vi "wb6OutputPlan.vi"() -> ()   [LabVIEW 2012]
uses:
  <vilib>/addons/database/Auxilliary.llb/DB Tools Cursor Type.ctl
  <vilib>/Utility/NIReport.llb/NI_report.lvclass
  <vilib>/addons/database/Connection.llb/DB Tools Open Connec (Path).vi
  <vilib>/addons/database/Connection.llb/Conn Execute.vi
  <vilib>/addons/database/Recordset.llb/Rec Fetch Recordset Data (R).vi
  <vilib>/addons/database/Recordset.llb/Rec Destroy - Connection.vi
  <vilib>/addons/database/Recordset.llb/Rec Fetch Integer Data (R).vi
  <vilib>/Utility/NIReport.llb/Append Text Table to Report (wrap).vi
  <vilib>/addons/database/_DB Variant To Data/Database Variant To Data.xnode
  <vilib>/addons/database/NI_Database_API.lvlib
  <vilib>/Utility/NIReport.llb/Excel/NI_Excel.lvclass
  <vilib>/addons/_office/NI_ReportGenerationToolkit.lvlib
  <vilib>/Utility/SMTP/NI_SMTPEmail.lvlib
panel:
  out "error out 2":errorcluster
  in  "text data":string[][](array[string])
  in  "text data 2":string[][](array[string])
  out "data 5":string
  out "concatenated string 8":string
  out "concatenated string 7":string
  out "concatenated string 6":string
  out "recordset data 2":variant[][](array[variant])
  out "data 4":string
  out "concatenated string 5":string
  out "error out 3":errorcluster
  out "data 2":string
  out "concatenated string":string
  out "concatenated string 3":string
  out "concatenated string 2":string
  out "recordset data":variant[][](array[variant])
  out "data 3":string
  out "concatenated string 4":string
  out "error out":errorcluster
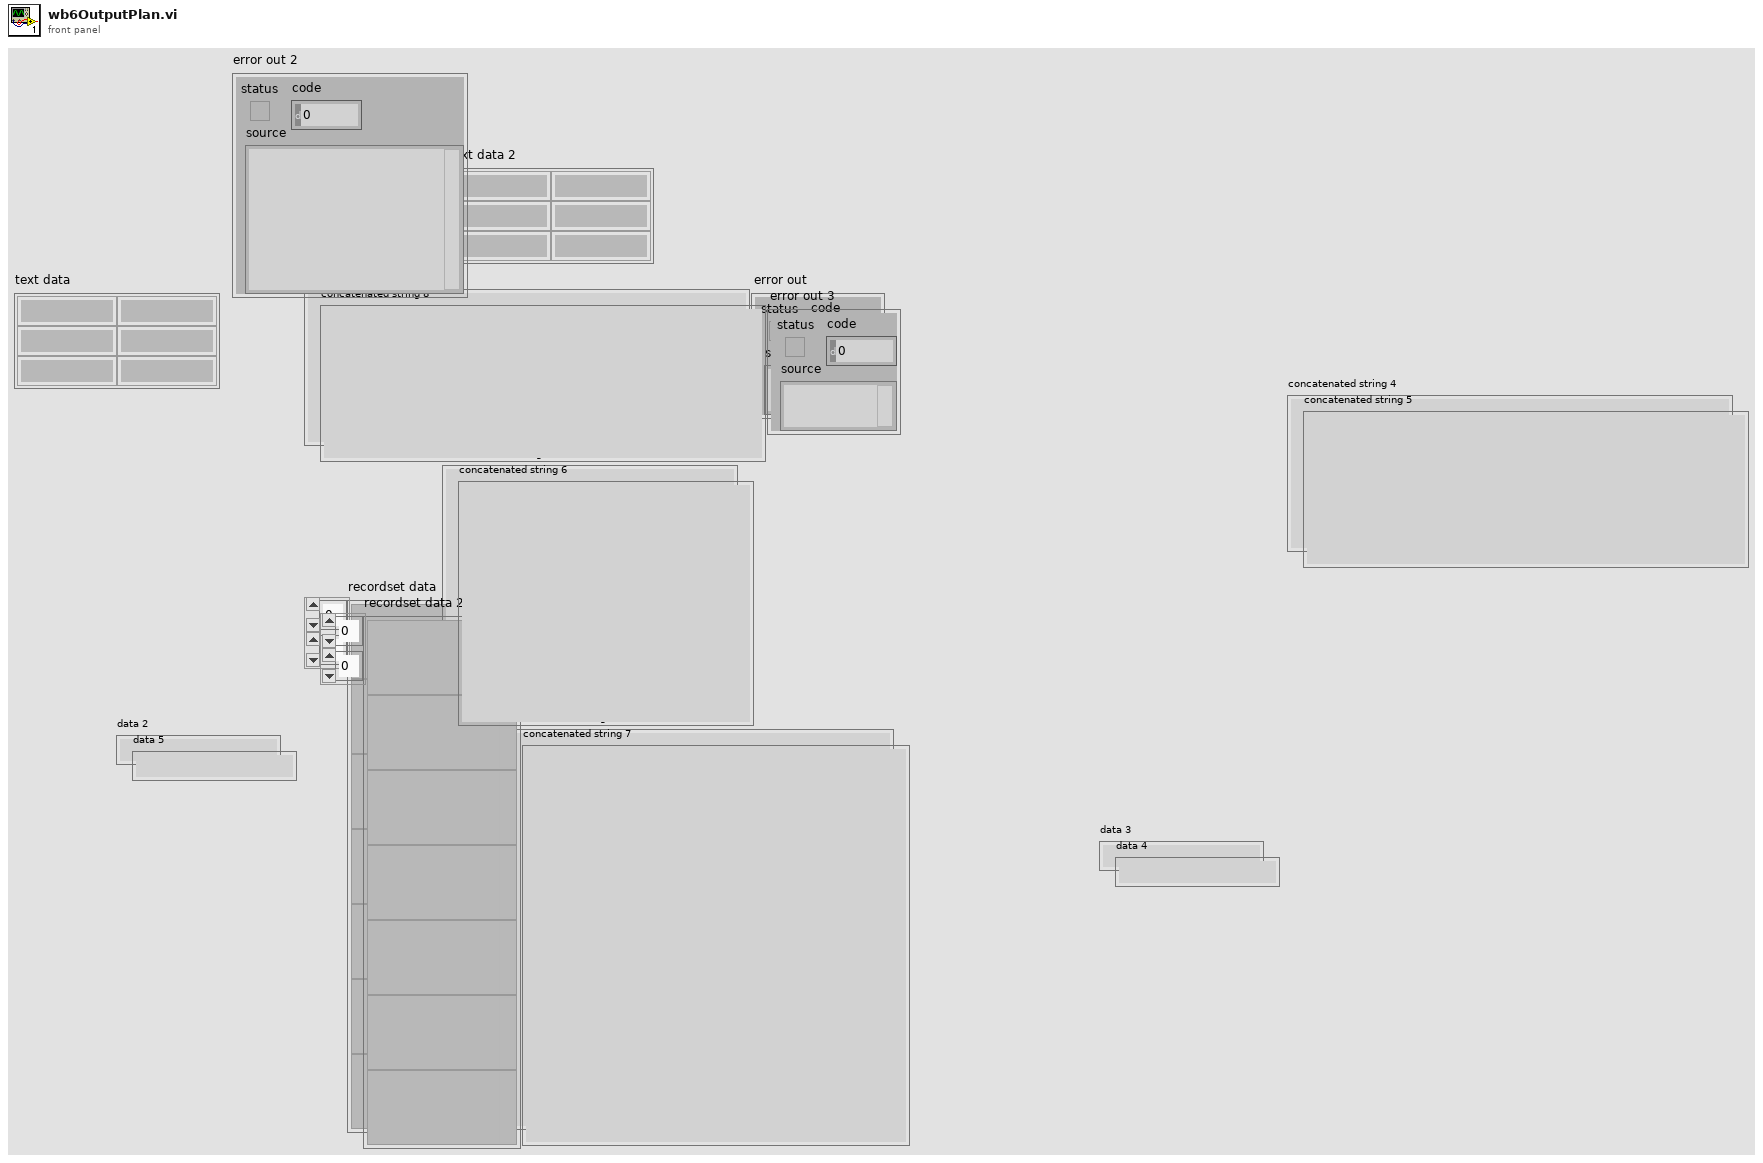
[diagram p1: front panel]
types:
  T1 = typedef "NI_Database_API.lvlib/DB Tools Cursor Type.ctl" = enum16{"forward-only", "keyset", "dynamic", "static"}
  T2 = typedef "NI_Database_API.lvlib/Conn ObjectReference.ctl" = refnum<k1>
  T3 = typedef "NI_Database_API.lvlib/Rec ObjectReference.ctl" = refnum<k1>
  T4 = enum16{"Standard Report", "HTML", "Word", "Excel"}
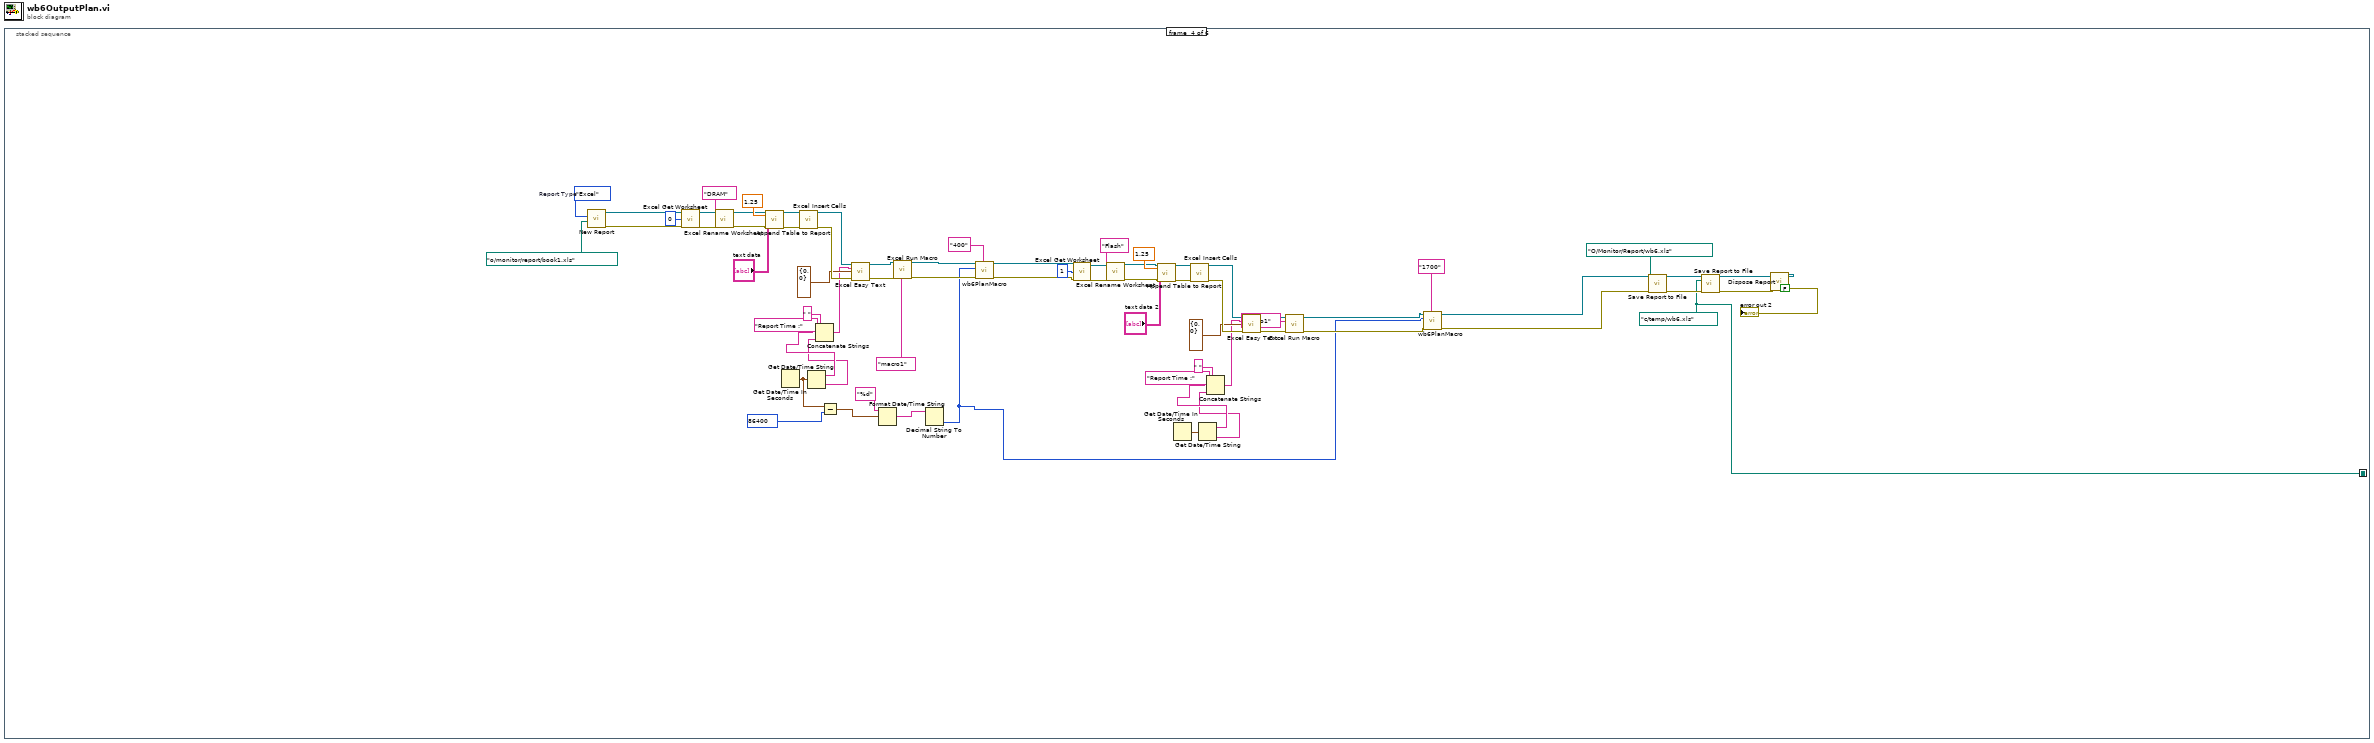
[diagram p0: block diagram]
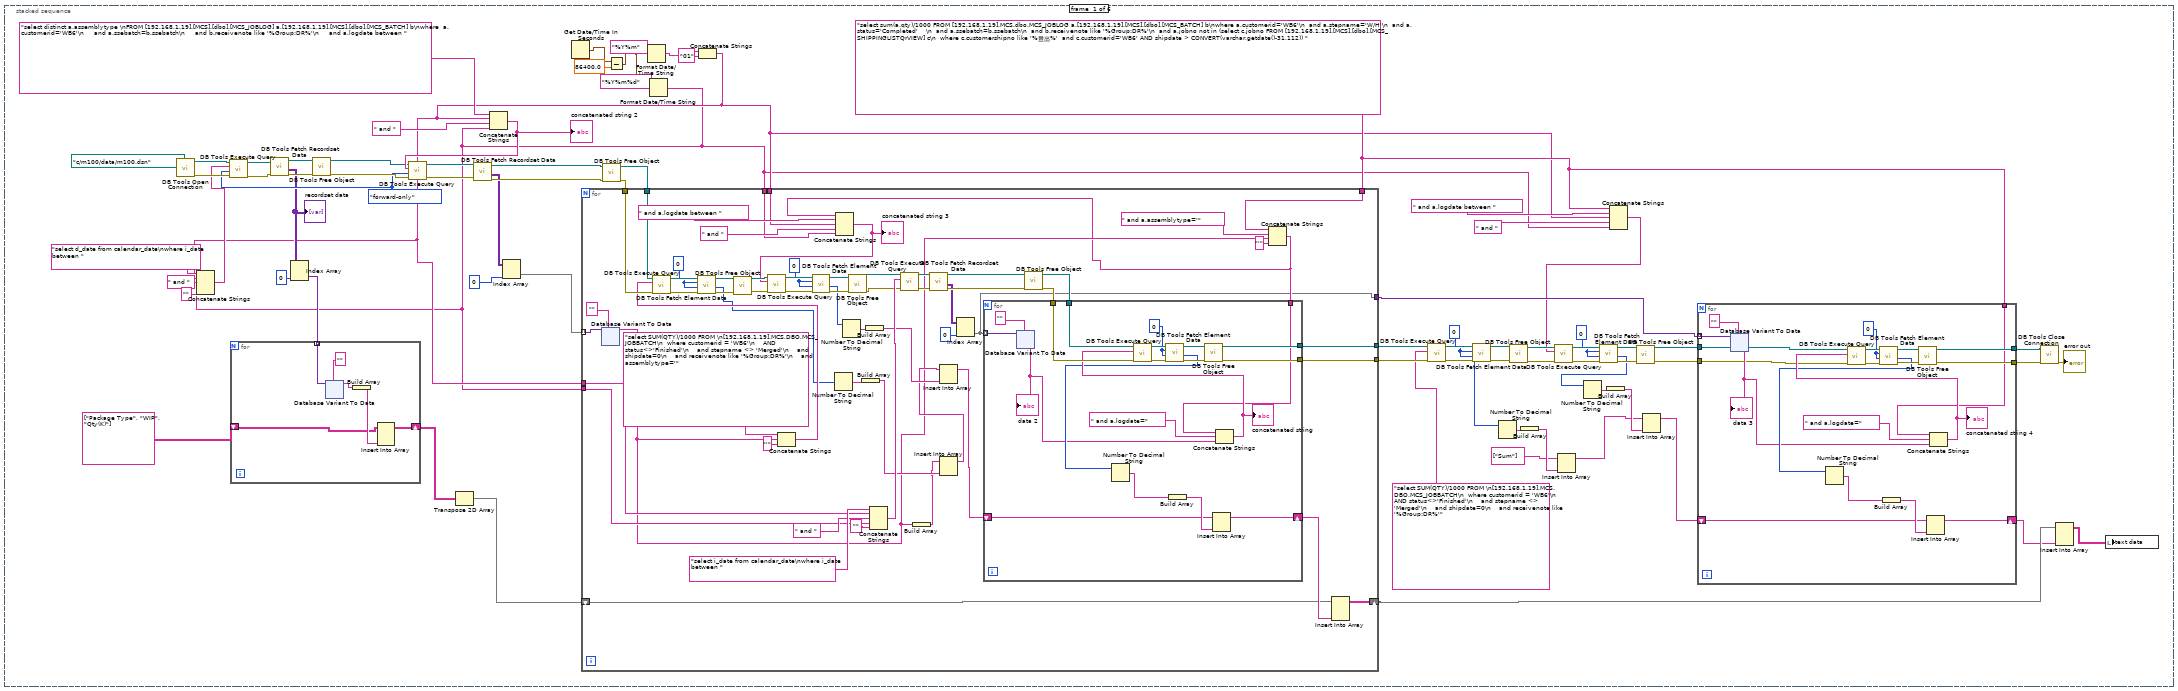
[diagram p2: hidden frame]
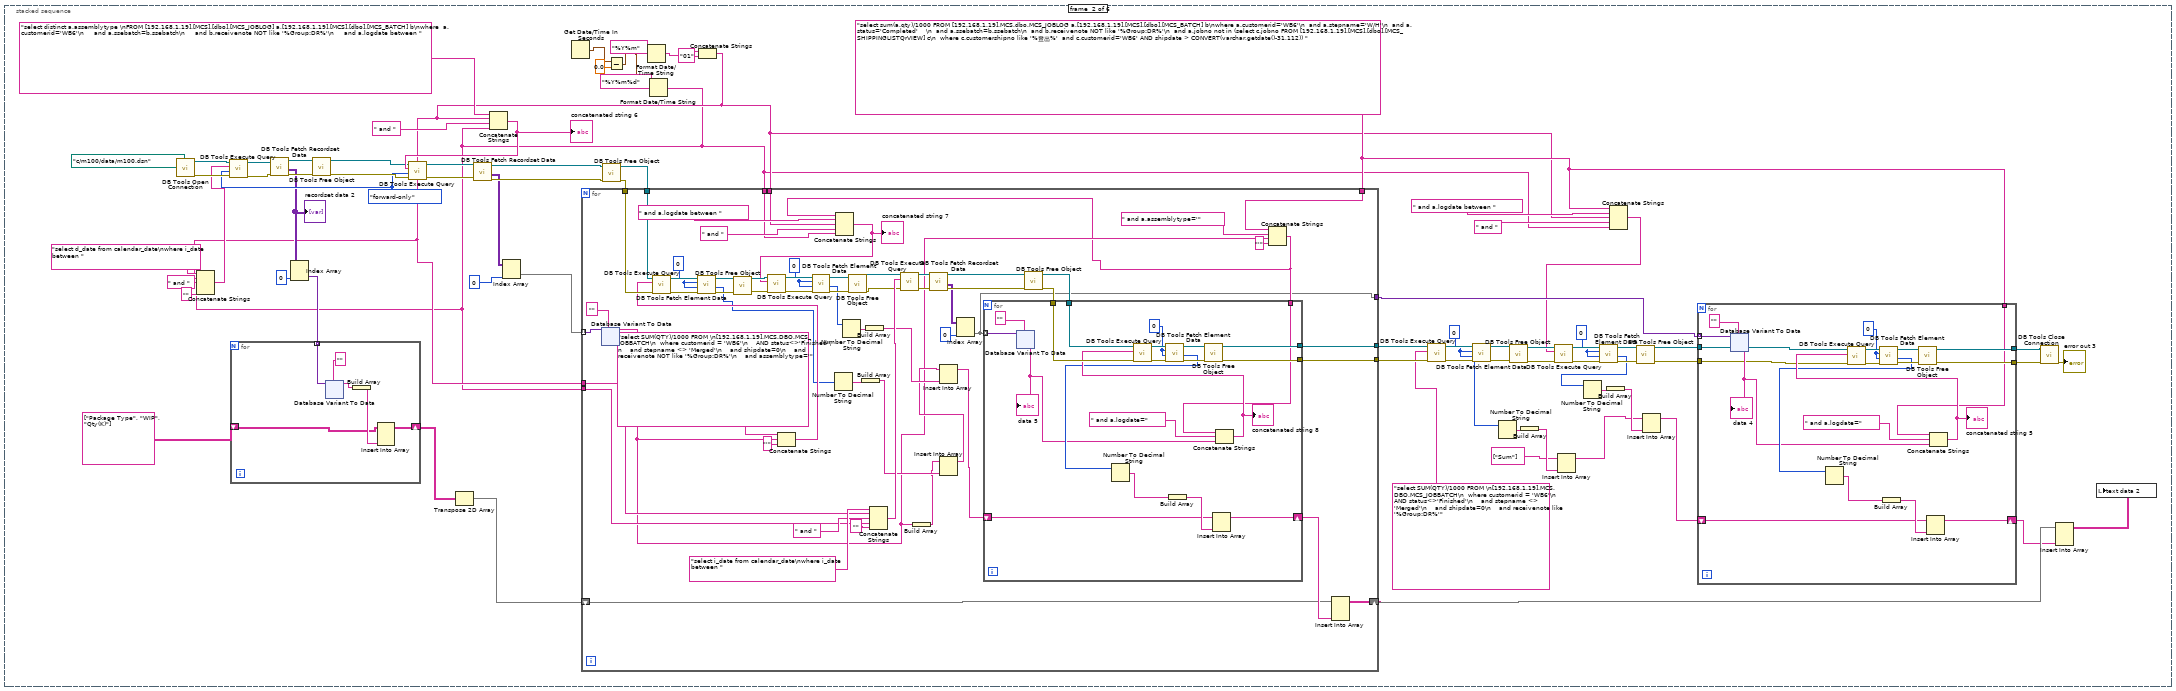
[diagram p3: hidden frame]
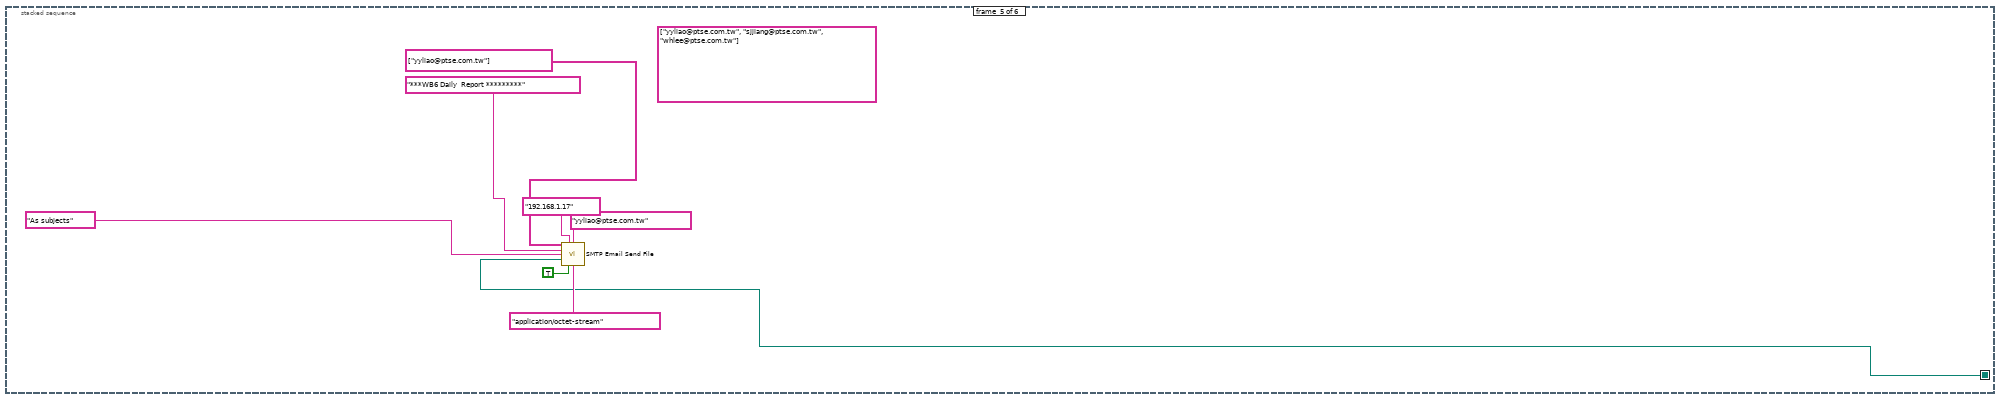
[diagram p5: hidden frame]
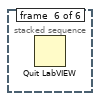
[diagram p6: hidden frame]
diagram:
  n1 = stacked-sequence {
    seq-local: [_ _ _ w641 _ _] -> [_ _ _ _ w697 _]
    frame #0 {
      w17 = 0
      w35 = 0
      w43 = DB_Tools_Cursor_Type."forward-only" ("cursor type")
      w5 = "select sum(a.qty)/1000 FROM [192.168.1.19].MCS.dbo.MCS_JOBLOG a,[192.168.1.19].[MCS].[dbo].[MCS_BATCH] b\nwhere a.customerid='WB6'\n  and a.stepname='W/H'\n  and a.status='Completed'    \n  and a.ssebatch=b.ssebatch\n  and b.receivenote like '%Group:DR%'\n  and a.jobno not in (select c.jobno FROM [192.168.1.19].[MCS].[dbo].[MCS_SHIPPINGLISTQrVIEW] c\n  where c.customershipno like '%登出%'  and c.customerid='WB6' AND shipdate > CONVERT(varchar,getdate()-31,112)) "
      n2 = call-poly <vilib>:"DB Tools Open Connection.vi"("connection information"=path "c:/m100/data/m100.dsn") -> ("error out"=w51:errorcluster, "connection reference"=w55:T2)  [unwired: 7 in]
      n3 = Get Date/Time In Seconds() -> (seconds since 1Jan1904=w68:timestamp)
      n4 = Subtract(x=w68, y=86400.0) -> (x-y=w63:timestamp)
      n5 = Format Date/Time String(time format string (%c)="%Y%m", seconds (now)=w63) -> (date/time string=w66:string)  [unwired: 1 in]
      n6 = Format Date/Time String(time format string (%c)="%Y%m%d", seconds (now)=w63) -> (date/time string=w3:string)  [unwired: 1 in]
      n7 = Concatenate Strings(w66, "01" ("string")) -> (w4:string)
      n8 = Concatenate Strings("select d_date from calendar_date\nwhere i_date between ", w4, " and " ("string"), w3, "" ("string")) -> (w44:string)
      n9 = call-poly <vilib>:"DB Tools Execute Query.vi"("error in (no error)"=w51, "cursor type"=w43, "SQL query"=w44, "connection reference"=w55) -> ("error out"=w50:errorcluster, "recordset reference"=w54:T3)  [unwired: 4 in]
      n10 = call-poly <vilib>:"DB Tools Fetch Recordset Data.vi"("error in (no error)"=w50, "recordset reference"=w54) -> ("error out"=w49:errorcluster, "recordset data"=w42:variant[][], "recordset reference out"=w53:T3)  [unwired: 3 in]
      "recordset data" <- w42
      n11 = Index Array(array=w42, index (col)=0 ("disabled index (col)")) -> (element=w41:variant[])  [unwired: 1 in]
      n12 = for {
        tunnel: w41 -> [w136] mode=indexing
        shift-right: [w132] -> w71
        shift-left: string[][] [["Package Type"], ["WIP"], ["Qty(K)"]] ("array") -> [w131]
        n13 = xnode "Database Variant To Data"("database variant"=w136, "type"="") -> ("data"=w134:string)  [unwired: 1 in, 1 out]
        n14 = Build Array(w134) -> (w133:string[])
        n15 = Insert Into Array(array=w131, new element=w133) -> (w132:string[][])  [unwired: 2 in]
      }
      n16 = call-poly <vilib>:"DB Tools Free Object.vi"("error in (no error)"=w49, "recordset reference"=w53) -> ("error out"=w48:errorcluster, "connection reference"=w52:T2)  [unwired: 8 in]
      n17 = Transpose 2D Array(2D array=w71) -> (transposed array=w70:string[][])
      n18 = Concatenate Strings("select distinct a.assemblytype \nFROM [192.168.1.19].[MCS].[dbo].[MCS_JOBLOG] a,[192.168.1.19].[MCS].[dbo].[MCS_BATCH] b\nwhere  a.customerid='WB6'\n     and a.ssebatch=b.ssebatch\n     and b.receivenote like '%Group:DR%'\n     and a.logdate between ", w4, " and " ("string"), w3) -> (w76:string)
      "concatenated string 2" <- w76
      n19 = call-poly <vilib>:"DB Tools Execute Query.vi"("error in (no error)"=w48, "cursor type"=w43, "SQL query"=w76, "connection reference"=w52) -> ("error out"=w61:errorcluster, "recordset reference"=w62:T3)  [unwired: 4 in]
      n20 = call-poly <vilib>:"DB Tools Fetch Recordset Data.vi"("error in (no error)"=w61, "recordset reference"=w62) -> ("error out"=w77:errorcluster, "recordset data"=w59:variant[][], "recordset reference out"=w78:T3)  [unwired: 3 in]
      n21 = Index Array(array=w59, index (col)=0 ("disabled index (col)")) -> (element=w75:variant[])  [unwired: 1 in]
      n22 = call-poly <vilib>:"DB Tools Free Object.vi"("error in (no error)"=w77, "recordset reference"=w78) -> ("error out"=w73:errorcluster, "connection reference"=w74:T2)  [unwired: 8 in]
      n23 = for {
        tunnel: w75 -> [w227] mode=indexing
        tunnel: w74 -> [w209]
        tunnel: w73 -> [w198]
        tunnel: [w214] -> w34
        tunnel: [w213] -> w33
        tunnel: w4 -> [w221]
        tunnel: w3 -> [w204]
        shift-right: [w211] -> w23
        shift-left: w70 -> [w210]
        tunnel: w5 -> [w177]
        tunnel: w4 -> [w175]
        tunnel: w3 -> [w173]
        tunnel: [w169] -> w27
        w191 = 0
        w201 = 0
        n24 = xnode "Database Variant To Data"("database variant"=w227, "type"="") -> ("data"=w178:string)  [unwired: 1 in, 1 out]
        n25 = Concatenate Strings("select SUM(QTY)/1000 FROM \n[192.168.1.19].MCS.DBO.MCS_JOBBATCH\n  where customerid = 'WB6'\n    AND status<>'Finished'\n    and stepname <> 'Merged'\n    and shipdate=0\n    and receivenote like '%Group:DR%'\n    and assemblytype='" ("SQL query"), w178, "'" ("string")) -> (w197:string)
        n26 = call-poly <vilib>:"DB Tools Execute Query.vi"("error in (no error)"=w198, "SQL query"=w197, "connection reference"=w209) -> ("error out"=w206:errorcluster, "recordset reference"=w208:T3)  [unwired: 5 in]
        n27 = call-poly <vilib>:"DB Tools Fetch Element Data.vi"("error in (no error)"=w206, "type"=w201, "column index"=w201, "recordset reference"=w208) -> ("error out"=w205:errorcluster, "data"=w196:i32, "recordset reference out"=w207:T3)  [unwired: 3 in]
        n28 = call-poly <vilib>:"DB Tools Free Object.vi"("error in (no error)"=w205, "recordset reference"=w207) -> ("error out"=w189:errorcluster, "connection reference"=w190:T2)  [unwired: 8 in]
        n29 = Number To Decimal String(number=w196) -> (decimal integer string=w200:string)  [unwired: 1 in]
        n30 = Build Array(w200) -> (w199:string[])
        n31 = Concatenate Strings("select i_date from calendar_date\nwhere i_date between ", w221, " and " ("string"), w204, "" ("string")) -> (w219:string)
        n32 = Build Array "Build Array"(w178) -> (w180:string[])
        n33 = Insert Into Array(array=w180, new element=w199) -> (w182:string[])  [unwired: 1 in]
        n34 = Concatenate Strings(w177, " and a.assemblytype='" ("string"), w178, "'" ("string")) -> (w171:string)
        n35 = Concatenate Strings(w171, " and a.logdate between " ("string"), w175, " and " ("string"), w173) -> (w172:string)
        "concatenated string 3" <- w172
        n36 = call-poly <vilib>:"DB Tools Execute Query.vi"("error in (no error)"=w189, "SQL query"=w172, "connection reference"=w190) -> ("error out"=w193:errorcluster, "recordset reference"=w195:T3)  [unwired: 5 in]
        n37 = call-poly <vilib>:"DB Tools Fetch Element Data.vi"("error in (no error)"=w193, "type"=w191, "column index"=w191, "recordset reference"=w195) -> ("error out"=w192:errorcluster, "data"=w184:i32, "recordset reference out"=w194:T3)  [unwired: 3 in]
        n38 = Number To Decimal String(number=w184) -> (decimal integer string=w185:string)  [unwired: 1 in]
        n39 = call-poly <vilib>:"DB Tools Free Object.vi"("error in (no error)"=w192, "recordset reference"=w194) -> ("error out"=w187:errorcluster, "connection reference"=w188:T2)  [unwired: 8 in]
        n40 = Build Array(w185) -> (w183:string[])
        n41 = call-poly <vilib>:"DB Tools Execute Query.vi"("error in (no error)"=w187, "SQL query"=w219, "connection reference"=w188) -> ("error out"=w224:errorcluster, "recordset reference"=w226:T3)  [unwired: 5 in]
        n42 = call-poly <vilib>:"DB Tools Fetch Recordset Data.vi"("error in (no error)"=w224, "recordset reference"=w226) -> ("error out"=w223:errorcluster, "recordset data"=w170:variant[][], "recordset reference out"=w225:T3)  [unwired: 3 in]
        n43 = Insert Into Array(array=w182, new element=w183) -> (w181:string[])  [unwired: 1 in]
        n44 = Index Array(array=w170, index (col)=0 ("disabled index (col)")) -> (element=w169:variant[])  [unwired: 1 in]
        n45 = call-poly <vilib>:"DB Tools Free Object.vi"("error in (no error)"=w223, "recordset reference"=w225) -> ("error out"=w215:errorcluster, "connection reference"=w216:T2)  [unwired: 8 in]
        n46 = for {
          tunnel: w169 -> [w248] mode=indexing
          tunnel: w216 -> [w242]
          tunnel: w215 -> [w241]
          tunnel: [w240] -> w214
          tunnel: [w239] -> w213
          shift-right: [w233] -> w212
          shift-left: w181 -> [w232]
          tunnel: w171 -> [w229]
          w236 = 0
          n47 = xnode "Database Variant To Data"("database variant"=w248, "type"="") -> ("data"=w230:string)  [unwired: 1 in, 1 out]
          "data 2" <- w230
          n48 = Concatenate Strings(w229, " and a.logdate=" ("string"), w230) -> (w237:string)
          "concatenated string" <- w237
          n49 = call-poly <vilib>:"DB Tools Execute Query.vi"("error in (no error)"=w241, "SQL query"=w237, "connection reference"=w242) -> ("error out"=w244:errorcluster, "recordset reference"=w246:T3)  [unwired: 5 in]
          n50 = call-poly <vilib>:"DB Tools Fetch Element Data.vi"("error in (no error)"=w244, "type"=w236, "column index"=w236, "recordset reference"=w246) -> ("error out"=w243:errorcluster, "data"=w235:i32, "recordset reference out"=w245:T3)  [unwired: 3 in]
          n51 = Number To Decimal String(number=w235) -> (decimal integer string=w231:string)  [unwired: 1 in]
          n52 = Build Array(w231) -> (w234:string[])
          n53 = call-poly <vilib>:"DB Tools Free Object.vi"("error in (no error)"=w243, "recordset reference"=w245) -> ("error out"=w239:errorcluster, "connection reference"=w240:T2)  [unwired: 8 in]
          n54 = Insert Into Array(array=w232, new element=w234) -> (w233:string[])  [unwired: 1 in]
        }
        n55 = Insert Into Array(array=w210, new element=w212) -> (w211:string[][])  [unwired: 2 in]
      }
      n56 = call-poly <vilib>:"DB Tools Execute Query.vi"("error in (no error)"=w33, "SQL query"="select SUM(QTY)/1000 FROM \n[192.168.1.19].MCS.DBO.MCS_JOBBATCH\n  where customerid = 'WB6'\n    AND status<>'Finished'\n    and stepname <> 'Merged'\n    and shipdate=0\n    and receivenote like '%Group:DR%'", "connection reference"=w34) -> ("error out"=w37:errorcluster, "recordset reference"=w39:T3)  [unwired: 5 in]
      n57 = call-poly <vilib>:"DB Tools Fetch Element Data.vi"("error in (no error)"=w37, "type"=w35, "column index"=w35, "recordset reference"=w39) -> ("error out"=w36:errorcluster, "data"=w30:i32, "recordset reference out"=w38:T3)  [unwired: 3 in]
      n58 = Number To Decimal String(number=w30) -> (decimal integer string=w31:string)  [unwired: 1 in]
      n59 = call-poly <vilib>:"DB Tools Free Object.vi"("error in (no error)"=w36, "recordset reference"=w38) -> ("error out"=w15:errorcluster, "connection reference"=w16:T2)  [unwired: 8 in]
      n60 = Build Array(w31) -> (w29:string[])
      n61 = Insert Into Array(array=string[] ["Sum"], new element=w29) -> (w9:string[])  [unwired: 1 in]
      n62 = Concatenate Strings(w5, " and a.logdate between " ("string"), w4, " and " ("string"), w3) -> (w2:string)
      n63 = call-poly <vilib>:"DB Tools Execute Query.vi"("error in (no error)"=w15, "SQL query"=w2, "connection reference"=w16) -> ("error out"=w19:errorcluster, "recordset reference"=w21:T3)  [unwired: 5 in]
      n64 = call-poly <vilib>:"DB Tools Fetch Element Data.vi"("error in (no error)"=w19, "type"=w17, "column index"=w17, "recordset reference"=w21) -> ("error out"=w18:errorcluster, "data"=w10:i32, "recordset reference out"=w20:T3)  [unwired: 3 in]
      n65 = Number To Decimal String(number=w10) -> (decimal integer string=w12:string)  [unwired: 1 in]
      n66 = Build Array(w12) -> (w11:string[])
      n67 = call-poly <vilib>:"DB Tools Free Object.vi"("error in (no error)"=w18, "recordset reference"=w20) -> ("error out"=w13:errorcluster, "connection reference"=w14:T2)  [unwired: 8 in]
      n68 = Insert Into Array(array=w9, new element=w11) -> (w8:string[])  [unwired: 1 in]
      n69 = for {
        tunnel: w27 -> [w81] mode=indexing
        tunnel: [w93] -> w26
        tunnel: [w92] -> w25
        shift-right: [w86] -> w22
        shift-left: w8 -> [w85]
        tunnel: w5 -> [w82]
        tunnel: w14 -> [w80]
        tunnel: w13 -> [w79]
        w89 = 0
        n70 = xnode "Database Variant To Data"("database variant"=w81, "type"="") -> ("data"=w83:string)  [unwired: 1 in, 1 out]
        "data 3" <- w83
        n71 = Concatenate Strings(w82, " and a.logdate=" ("string"), w83) -> (w90:string)
        "concatenated string 4" <- w90
        n72 = call-poly <vilib>:"DB Tools Execute Query.vi"("error in (no error)"=w79, "SQL query"=w90, "connection reference"=w80) -> ("error out"=w95:errorcluster, "recordset reference"=w97:T3)  [unwired: 5 in]
        n73 = call-poly <vilib>:"DB Tools Fetch Element Data.vi"("error in (no error)"=w95, "type"=w89, "column index"=w89, "recordset reference"=w97) -> ("error out"=w94:errorcluster, "data"=w88:i32, "recordset reference out"=w96:T3)  [unwired: 3 in]
        n74 = Number To Decimal String(number=w88) -> (decimal integer string=w84:string)  [unwired: 1 in]
        n75 = Build Array(w84) -> (w87:string[])
        n76 = call-poly <vilib>:"DB Tools Free Object.vi"("error in (no error)"=w94, "recordset reference"=w96) -> ("error out"=w92:errorcluster, "connection reference"=w93:T2)  [unwired: 8 in]
        n77 = Insert Into Array(array=w85, new element=w87) -> (w86:string[])  [unwired: 1 in]
      }
      n78 = call <vilib>:"DB Tools Close Connection.vi"("error in (no error)"=w25, "connection reference"=w26) -> ("error out"=→"error out":errorcluster)  [unwired: 5 in]
      n79 = Insert Into Array(array=w23, new element=w22) -> (w1:string[][])  [unwired: 2 in]
      n80 = local write "text data"(w1) -> ()
    }
    frame #1 {
      w329 = 0
      w347 = 0
      w355 = DB_Tools_Cursor_Type."forward-only" ("cursor type")
      w317 = "select sum(a.qty)/1000 FROM [192.168.1.19].MCS.dbo.MCS_JOBLOG a,[192.168.1.19].[MCS].[dbo].[MCS_BATCH] b\nwhere a.customerid='WB6'\n  and a.stepname='W/H'\n  and a.status='Completed'    \n  and a.ssebatch=b.ssebatch\n  and b.receivenote NOT like '%Group:DR%'\n  and a.jobno not in (select c.jobno FROM [192.168.1.19].[MCS].[dbo].[MCS_SHIPPINGLISTQrVIEW] c\n  where c.customershipno like '%登出%'  and c.customerid='WB6' AND shipdate > CONVERT(varchar,getdate()-31,112)) "
      n81 = call-poly <vilib>:"DB Tools Open Connection.vi"("connection information"=path "c:/m100/data/m100.dsn") -> ("error out"=w363:errorcluster, "connection reference"=w367:T2)  [unwired: 7 in]
      n82 = Get Date/Time In Seconds() -> (seconds since 1Jan1904=w380:timestamp)
      n83 = Subtract(x=w380, y=0.0) -> (x-y=w375:timestamp)
      n84 = Format Date/Time String(time format string (%c)="%Y%m", seconds (now)=w375) -> (date/time string=w378:string)  [unwired: 1 in]
      n85 = Format Date/Time String(time format string (%c)="%Y%m%d", seconds (now)=w375) -> (date/time string=w315:string)  [unwired: 1 in]
      n86 = Concatenate Strings(w378, "01" ("string")) -> (w316:string)
      n87 = Concatenate Strings("select d_date from calendar_date\nwhere i_date between ", w316, " and " ("string"), w315, "" ("string")) -> (w356:string)
      n88 = call-poly <vilib>:"DB Tools Execute Query.vi"("error in (no error)"=w363, "cursor type"=w355, "SQL query"=w356, "connection reference"=w367) -> ("error out"=w362:errorcluster, "recordset reference"=w366:T3)  [unwired: 4 in]
      n89 = call-poly <vilib>:"DB Tools Fetch Recordset Data.vi"("error in (no error)"=w362, "recordset reference"=w366) -> ("error out"=w361:errorcluster, "recordset data"=w354:variant[][], "recordset reference out"=w365:T3)  [unwired: 3 in]
      "recordset data 2" <- w354
      n90 = Index Array(array=w354, index (col)=0 ("disabled index (col)")) -> (element=w353:variant[])  [unwired: 1 in]
      n91 = for {
        tunnel: w353 -> [w448] mode=indexing
        shift-right: [w444] -> w383
        shift-left: string[][] [["Package Type"], ["WIP"], ["Qty(K)"]] ("array") -> [w443]
        n92 = xnode "Database Variant To Data"("database variant"=w448, "type"="") -> ("data"=w446:string)  [unwired: 1 in, 1 out]
        n93 = Build Array(w446) -> (w445:string[])
        n94 = Insert Into Array(array=w443, new element=w445) -> (w444:string[][])  [unwired: 2 in]
      }
      n95 = call-poly <vilib>:"DB Tools Free Object.vi"("error in (no error)"=w361, "recordset reference"=w365) -> ("error out"=w360:errorcluster, "connection reference"=w364:T2)  [unwired: 8 in]
      n96 = Transpose 2D Array(2D array=w383) -> (transposed array=w382:string[][])
      n97 = Concatenate Strings("select distinct a.assemblytype \nFROM [192.168.1.19].[MCS].[dbo].[MCS_JOBLOG] a,[192.168.1.19].[MCS].[dbo].[MCS_BATCH] b\nwhere  a.customerid='WB6'\n     and a.ssebatch=b.ssebatch\n     and b.receivenote NOT like '%Group:DR%'\n     and a.logdate between ", w316, " and " ("string"), w315) -> (w388:string)
      "concatenated string 6" <- w388
      n98 = call-poly <vilib>:"DB Tools Execute Query.vi"("error in (no error)"=w360, "cursor type"=w355, "SQL query"=w388, "connection reference"=w364) -> ("error out"=w373:errorcluster, "recordset reference"=w374:T3)  [unwired: 4 in]
      n99 = call-poly <vilib>:"DB Tools Fetch Recordset Data.vi"("error in (no error)"=w373, "recordset reference"=w374) -> ("error out"=w389:errorcluster, "recordset data"=w371:variant[][], "recordset reference out"=w390:T3)  [unwired: 3 in]
      n100 = Index Array(array=w371, index (col)=0 ("disabled index (col)")) -> (element=w387:variant[])  [unwired: 1 in]
      n101 = call-poly <vilib>:"DB Tools Free Object.vi"("error in (no error)"=w389, "recordset reference"=w390) -> ("error out"=w385:errorcluster, "connection reference"=w386:T2)  [unwired: 8 in]
      n102 = for {
        tunnel: w387 -> [w539] mode=indexing
        tunnel: w386 -> [w521]
        tunnel: w385 -> [w510]
        tunnel: [w526] -> w346
        tunnel: [w525] -> w345
        tunnel: w316 -> [w533]
        tunnel: w315 -> [w516]
        shift-right: [w523] -> w335
        shift-left: w382 -> [w522]
        tunnel: w317 -> [w489]
        tunnel: w316 -> [w487]
        tunnel: w315 -> [w485]
        tunnel: [w481] -> w339
        w503 = 0
        w513 = 0
        n103 = xnode "Database Variant To Data"("database variant"=w539, "type"="") -> ("data"=w490:string)  [unwired: 1 in, 1 out]
        n104 = Concatenate Strings("select SUM(QTY)/1000 FROM \n[192.168.1.19].MCS.DBO.MCS_JOBBATCH\n  where customerid = 'WB6'\n    AND status<>'Finished'\n    and stepname <> 'Merged'\n    and shipdate=0\n    and receivenote NOT like '%Group:DR%'\n    and assemblytype='" ("SQL query"), w490, "'" ("string")) -> (w509:string)
        n105 = call-poly <vilib>:"DB Tools Execute Query.vi"("error in (no error)"=w510, "SQL query"=w509, "connection reference"=w521) -> ("error out"=w518:errorcluster, "recordset reference"=w520:T3)  [unwired: 5 in]
        n106 = call-poly <vilib>:"DB Tools Fetch Element Data.vi"("error in (no error)"=w518, "type"=w513, "column index"=w513, "recordset reference"=w520) -> ("error out"=w517:errorcluster, "data"=w508:i32, "recordset reference out"=w519:T3)  [unwired: 3 in]
        n107 = call-poly <vilib>:"DB Tools Free Object.vi"("error in (no error)"=w517, "recordset reference"=w519) -> ("error out"=w501:errorcluster, "connection reference"=w502:T2)  [unwired: 8 in]
        n108 = Number To Decimal String(number=w508) -> (decimal integer string=w512:string)  [unwired: 1 in]
        n109 = Build Array(w512) -> (w511:string[])
        n110 = Concatenate Strings("select i_date from calendar_date\nwhere i_date between ", w533, " and " ("string"), w516, "" ("string")) -> (w531:string)
        n111 = Build Array "Build Array"(w490) -> (w492:string[])
        n112 = Insert Into Array(array=w492, new element=w511) -> (w494:string[])  [unwired: 1 in]
        n113 = Concatenate Strings(w489, " and a.assemblytype='" ("string"), w490, "'" ("string")) -> (w483:string)
        n114 = Concatenate Strings(w483, " and a.logdate between " ("string"), w487, " and " ("string"), w485) -> (w484:string)
        "concatenated string 7" <- w484
        n115 = call-poly <vilib>:"DB Tools Execute Query.vi"("error in (no error)"=w501, "SQL query"=w484, "connection reference"=w502) -> ("error out"=w505:errorcluster, "recordset reference"=w507:T3)  [unwired: 5 in]
        n116 = call-poly <vilib>:"DB Tools Fetch Element Data.vi"("error in (no error)"=w505, "type"=w503, "column index"=w503, "recordset reference"=w507) -> ("error out"=w504:errorcluster, "data"=w496:i32, "recordset reference out"=w506:T3)  [unwired: 3 in]
        n117 = Number To Decimal String(number=w496) -> (decimal integer string=w497:string)  [unwired: 1 in]
        n118 = call-poly <vilib>:"DB Tools Free Object.vi"("error in (no error)"=w504, "recordset reference"=w506) -> ("error out"=w499:errorcluster, "connection reference"=w500:T2)  [unwired: 8 in]
        n119 = Build Array(w497) -> (w495:string[])
        n120 = call-poly <vilib>:"DB Tools Execute Query.vi"("error in (no error)"=w499, "SQL query"=w531, "connection reference"=w500) -> ("error out"=w536:errorcluster, "recordset reference"=w538:T3)  [unwired: 5 in]
        n121 = call-poly <vilib>:"DB Tools Fetch Recordset Data.vi"("error in (no error)"=w536, "recordset reference"=w538) -> ("error out"=w535:errorcluster, "recordset data"=w482:variant[][], "recordset reference out"=w537:T3)  [unwired: 3 in]
        n122 = Insert Into Array(array=w494, new element=w495) -> (w493:string[])  [unwired: 1 in]
        n123 = Index Array(array=w482, index (col)=0 ("disabled index (col)")) -> (element=w481:variant[])  [unwired: 1 in]
        n124 = call-poly <vilib>:"DB Tools Free Object.vi"("error in (no error)"=w535, "recordset reference"=w537) -> ("error out"=w527:errorcluster, "connection reference"=w528:T2)  [unwired: 8 in]
        n125 = for {
          tunnel: w481 -> [w560] mode=indexing
          tunnel: w528 -> [w554]
          tunnel: w527 -> [w553]
          tunnel: [w552] -> w526
          tunnel: [w551] -> w525
          shift-right: [w545] -> w524
          shift-left: w493 -> [w544]
          tunnel: w483 -> [w541]
          w548 = 0
          n126 = xnode "Database Variant To Data"("database variant"=w560, "type"="") -> ("data"=w542:string)  [unwired: 1 in, 1 out]
          "data 5" <- w542
          n127 = Concatenate Strings(w541, " and a.logdate=" ("string"), w542) -> (w549:string)
          "concatenated string 8" <- w549
          n128 = call-poly <vilib>:"DB Tools Execute Query.vi"("error in (no error)"=w553, "SQL query"=w549, "connection reference"=w554) -> ("error out"=w556:errorcluster, "recordset reference"=w558:T3)  [unwired: 5 in]
          n129 = call-poly <vilib>:"DB Tools Fetch Element Data.vi"("error in (no error)"=w556, "type"=w548, "column index"=w548, "recordset reference"=w558) -> ("error out"=w555:errorcluster, "data"=w547:i32, "recordset reference out"=w557:T3)  [unwired: 3 in]
          n130 = Number To Decimal String(number=w547) -> (decimal integer string=w543:string)  [unwired: 1 in]
          n131 = Build Array(w543) -> (w546:string[])
          n132 = call-poly <vilib>:"DB Tools Free Object.vi"("error in (no error)"=w555, "recordset reference"=w557) -> ("error out"=w551:errorcluster, "connection reference"=w552:T2)  [unwired: 8 in]
          n133 = Insert Into Array(array=w544, new element=w546) -> (w545:string[])  [unwired: 1 in]
        }
        n134 = Insert Into Array(array=w522, new element=w524) -> (w523:string[][])  [unwired: 2 in]
      }
      n135 = call-poly <vilib>:"DB Tools Execute Query.vi"("error in (no error)"=w345, "SQL query"="select SUM(QTY)/1000 FROM \n[192.168.1.19].MCS.DBO.MCS_JOBBATCH\n  where customerid = 'WB6'\n    AND status<>'Finished'\n    and stepname <> 'Merged'\n    and shipdate=0\n    and receivenote like '%Group:DR%'", "connection reference"=w346) -> ("error out"=w349:errorcluster, "recordset reference"=w351:T3)  [unwired: 5 in]
      n136 = call-poly <vilib>:"DB Tools Fetch Element Data.vi"("error in (no error)"=w349, "type"=w347, "column index"=w347, "recordset reference"=w351) -> ("error out"=w348:errorcluster, "data"=w342:i32, "recordset reference out"=w350:T3)  [unwired: 3 in]
      n137 = Number To Decimal String(number=w342) -> (decimal integer string=w343:string)  [unwired: 1 in]
      n138 = call-poly <vilib>:"DB Tools Free Object.vi"("error in (no error)"=w348, "recordset reference"=w350) -> ("error out"=w327:errorcluster, "connection reference"=w328:T2)  [unwired: 8 in]
      n139 = Build Array(w343) -> (w341:string[])
      n140 = Insert Into Array(array=string[] ["Sum"], new element=w341) -> (w321:string[])  [unwired: 1 in]
      n141 = Concatenate Strings(w317, " and a.logdate between " ("string"), w316, " and " ("string"), w315) -> (w314:string)
      n142 = call-poly <vilib>:"DB Tools Execute Query.vi"("error in (no error)"=w327, "SQL query"=w314, "connection reference"=w328) -> ("error out"=w331:errorcluster, "recordset reference"=w333:T3)  [unwired: 5 in]
      n143 = call-poly <vilib>:"DB Tools Fetch Element Data.vi"("error in (no error)"=w331, "type"=w329, "column index"=w329, "recordset reference"=w333) -> ("error out"=w330:errorcluster, "data"=w322:i32, "recordset reference out"=w332:T3)  [unwired: 3 in]
      n144 = Number To Decimal String(number=w322) -> (decimal integer string=w324:string)  [unwired: 1 in]
      n145 = Build Array(w324) -> (w323:string[])
      n146 = call-poly <vilib>:"DB Tools Free Object.vi"("error in (no error)"=w330, "recordset reference"=w332) -> ("error out"=w325:errorcluster, "connection reference"=w326:T2)  [unwired: 8 in]
      n147 = Insert Into Array(array=w321, new element=w323) -> (w320:string[])  [unwired: 1 in]
      n148 = for {
        tunnel: w339 -> [w393] mode=indexing
        tunnel: [w405] -> w338
        tunnel: [w404] -> w337
        shift-right: [w398] -> w334
        shift-left: w320 -> [w397]
        tunnel: w317 -> [w394]
        tunnel: w326 -> [w392]
        tunnel: w325 -> [w391]
        w401 = 0
        n149 = xnode "Database Variant To Data"("database variant"=w393, "type"="") -> ("data"=w395:string)  [unwired: 1 in, 1 out]
        "data 4" <- w395
        n150 = Concatenate Strings(w394, " and a.logdate=" ("string"), w395) -> (w402:string)
        "concatenated string 5" <- w402
        n151 = call-poly <vilib>:"DB Tools Execute Query.vi"("error in (no error)"=w391, "SQL query"=w402, "connection reference"=w392) -> ("error out"=w407:errorcluster, "recordset reference"=w409:T3)  [unwired: 5 in]
        n152 = call-poly <vilib>:"DB Tools Fetch Element Data.vi"("error in (no error)"=w407, "type"=w401, "column index"=w401, "recordset reference"=w409) -> ("error out"=w406:errorcluster, "data"=w400:i32, "recordset reference out"=w408:T3)  [unwired: 3 in]
        n153 = Number To Decimal String(number=w400) -> (decimal integer string=w396:string)  [unwired: 1 in]
        n154 = Build Array(w396) -> (w399:string[])
        n155 = call-poly <vilib>:"DB Tools Free Object.vi"("error in (no error)"=w406, "recordset reference"=w408) -> ("error out"=w404:errorcluster, "connection reference"=w405:T2)  [unwired: 8 in]
        n156 = Insert Into Array(array=w397, new element=w399) -> (w398:string[])  [unwired: 1 in]
      }
      n157 = call <vilib>:"DB Tools Close Connection.vi"("error in (no error)"=w337, "connection reference"=w338) -> ("error out"=→"error out 3":errorcluster)  [unwired: 5 in]
      n158 = Insert Into Array(array=w335, new element=w334) -> (w313:string[][])  [unwired: 2 in]
      n159 = local write "text data 2"(w313) -> ()
    }
    frame #2 {
      # "select a.customerid,a.assemblytype,a.producttype,a.jobno,a.qty,a.logdate,a.logtime FROM [192.168.1.19].MCS.dbo.MCS_JOBLOG a,[192.168.1.19].[MCS].[dbo].[MCS_BATCH] b\nwhere a.customerid='WB6'\n  and a.stepname='W/H'\n  and a.status='Completed'    \n  and a.ssebatch=b.ssebatch\n  and b.receivenote NOT like '%Group:DR%'\n  and a.jobno not in (select c.jobno FROM [192.168.1.19].[MCS].[dbo].[MCS_SHIPPINGLISTQrVIEW] c\n  where c.customershipno like '%登出%'  and c.customerid='WB6' AND shipdate > CONVERT(varchar,getdate()-31,112)) \n  and a.logdate =20150921"
    }
    frame #3 {
      w641 = path "c:/temp/wb6.xls" ("report file path")
      w695 = T4."Excel"  # Report Type
      n160 = call <vilib>:"New Report.vi"("report type"=w695, "template (empty)"=path "o:/monitor/report/book1.xls" ("Report Template")) -> ("report out"=w690:refnum<class "NI_report.lvclass">, "error out"=w689:errorcluster)  [unwired: 12 in]
      n161 = call <vilib>:"Excel Get Worksheet.vi"("report in"=w690, "worksheet index (0)"=0, "error in (no error)"=w689) -> ("report out"=w687:refnum<class "NI_report.lvclass">, "error out"=w685:errorcluster)  [unwired: 11 in]
      n162 = call <vilib>:"Excel Rename Worksheet.vi"("report in"=w687, "worksheet name (\"\")"="DRAM" ("worksheet name (\"\")"), "error in (no error)"=w685) -> ("report out"=w686:refnum<class "NI_report.lvclass">, "error out"=w684:errorcluster)  [unwired: 11 in]
      n163 = call-poly <vilib>:"Append Table to Report.vi"("report in"=w686, "column width (1)"=1.25, "text data"="text data", "error in (no error)"=w684) -> ("report out"=w692:refnum<class "NI_report.lvclass">, "error out"=w691:errorcluster)  [unwired: 8 in, 2 out]
      n164 = Get Date/Time In Seconds() -> (seconds since 1Jan1904=w635:timestamp)
      n165 = call <vilib>:"Excel Insert Cells.vi"("report in"=w692, "error in (no error)"=w691) -> ("report out"=w682:refnum<class "NI_report.lvclass">, "error out"=w681:errorcluster)  [unwired: 12 in]
      n166 = Get Date/Time String(seconds (now)=w635) -> (date string=w678:string, time string=w676:string)  [unwired: 2 in]
      n167 = Concatenate Strings("Report Time :" ("string"), w678, " " ("string"), w676) -> (w675:string)
      n168 = Subtract(x=w635, y=86400) -> (x-y=w633:timestamp)
      n169 = call <vilib>:"Excel Easy Text.vi"("report in"=w682, "text"=w675, "start (-1, -1)"=cluster{"row":i32, "column":i32} {"row"=0, "column"=0} ("end (-1, -1)"), "error in (no error)"=w681) -> ("report out"=w643:refnum<class "NI_report.lvclass">, "error out"=w642:errorcluster)  [unwired: 7 in, 3 out]
      n170 = Format Date/Time String(time format string (%c)="%d", seconds (now)=w633) -> (date/time string=w631:string)  [unwired: 1 in]
      n171 = call <vilib>:"Excel Run Macro.vi"("report in"=w643, "macro name"="macro1", "error in (no error)"=w642) -> ("report out"=w640:refnum<class "NI_report.lvclass">, "error out"=w639:errorcluster)  [unwired: 10 in, 1 out]
      n172 = Decimal String To Number(string=w631) -> (number=w625:i32)  [unwired: 2 in, 1 out]
      n173 = call "wb6PlanMacro.vi"("TargetQty"="400", "error in (no error)"=w639, "Days"=w625, "report in"=w640) -> ("error out"=w637:errorcluster, "report out"=w638:refnum<class "NI_report.lvclass">)  [unwired: 6 in]
      n174 = call <vilib>:"Excel Get Worksheet.vi"("report in"=w638, "worksheet index (0)"=1, "error in (no error)"=w637) -> ("report out"=w662:refnum<class "NI_report.lvclass">, "error out"=w660:errorcluster)  [unwired: 11 in]
      n175 = call <vilib>:"Excel Rename Worksheet.vi"("report in"=w662, "worksheet name (\"\")"="Flash" ("worksheet name (\"\")"), "error in (no error)"=w660) -> ("report out"=w661:refnum<class "NI_report.lvclass">, "error out"=w659:errorcluster)  [unwired: 11 in]
      n176 = call-poly <vilib>:"Append Table to Report.vi"("report in"=w661, "column width (1)"=1.25, "text data"="text data 2", "error in (no error)"=w659) -> ("report out"=w665:refnum<class "NI_report.lvclass">, "error out"=w664:errorcluster)  [unwired: 8 in, 2 out]
      n177 = Get Date/Time In Seconds() -> (seconds since 1Jan1904=w653:timestamp)
      n178 = call <vilib>:"Excel Insert Cells.vi"("report in"=w665, "error in (no error)"=w664) -> ("report out"=w657:refnum<class "NI_report.lvclass">, "error out"=w656:errorcluster)  [unwired: 12 in]
      n179 = Get Date/Time String(seconds (now)=w653) -> (date string=w652:string, time string=w650:string)  [unwired: 2 in]
      n180 = Concatenate Strings("Report Time :" ("string"), w652, " " ("string"), w650) -> (w649:string)
      n181 = call <vilib>:"Excel Easy Text.vi"("report in"=w657, "text"=w649, "start (-1, -1)"=cluster{"row":i32, "column":i32} {"row"=0, "column"=0} ("end (-1, -1)"), "error in (no error)"=w656) -> ("report out"=w646:refnum<class "NI_report.lvclass">, "error out"=w647:errorcluster)  [unwired: 7 in, 3 out]
      n182 = call <vilib>:"Excel Run Macro.vi"("report in"=w646, "macro name"="macro1", "error in (no error)"=w647) -> ("report out"=w629:refnum<class "NI_report.lvclass">, "error out"=w627:errorcluster)  [unwired: 10 in, 1 out]
      n183 = call "wb6PlanMacro.vi"("TargetQty"="1700", "error in (no error)"=w627, "Days"=w625, "report in"=w629) -> ("error out"=w626:errorcluster, "report out"=w628:refnum<class "NI_report.lvclass">)  [unwired: 6 in]
      n184 = call-dynamic "Save Report to File.vi"("report in"=w628, "report file path"=path "O:/Monitor/Report/wb6.xls", "error in (no error)"=w626) -> ("report out"=w671:refnum<class "NI_report.lvclass">, "error out"=w669:errorcluster)  [unwired: 11 in]
      n185 = call-dynamic "Save Report to File.vi"("report in"=w671, "report file path"=w641, "error in (no error)"=w669) -> ("report out"=w670:refnum<class "NI_report.lvclass">, "error out"=w668:errorcluster)  [unwired: 11 in]
      n186 = call-dynamic "Dispose Report.vi"("report in"=w670, "save changes? (F)"=FALSE, "error in (no error)"=w668) -> ("error out"=→"error out 2":errorcluster)  [unwired: 12 in]
    }
    frame #4 {
      (unwired) string[] ["yyliao@ptse.com.tw", "sjjiang@ptse.com.tw", "whlee@ptse.com.tw"] ("recipients")
      n187 = call <vilib>:"SMTP Email Send File.vi"("recipients"=string[] ["yyliao@ptse.com.tw"], "mail server"="192.168.1.17", "return address"="yyliao@ptse.com.tw", "subject ([No Subject])"="***WB6 Daily  Report *********", "message"="As subjects", "file path"=w697, "binary? (F)"=TRUE, "MIME content-type (application/octet-stream)"="application/octet-stream") -> ()  [unwired: 6 in, 2 out]
    }
    frame #5 {
      n188 = Quit LabVIEW() -> ()  [unwired: 1 in]
    }
  }
